vi "Handle Error.vi"(8 "error in (no error)":errorcluster, 11 "UI Actor in":refnum<class "UI Actor.lvclass">) -> (0 "error out":errorcluster, 2 "stop actor?":bool=TRUE, 3 "UI Actor out":refnum<class "UI Actor.lvclass">)   [LabVIEW 2024, in "UI Actor.lvlib" / "UI Actor.lvclass"]
doc: "<p>(<strong>Filename</strong>: <span class=\"dnl\">Actor Framework.lvlib:Actor.lvclass:Handle Error.vi</span>)</p>\n<p>Defines how the actor handles an error that occurred while processing a message. By default, this method does nothing except stop the actor.</p>"
uses:
  UI Actor.lvclass
  UI Actor.lvclass/UI Actor.ctl
  <vilib>/MGI/Panel Manager/Panel Actor/Panel Actor/Panel Actor.lvclass
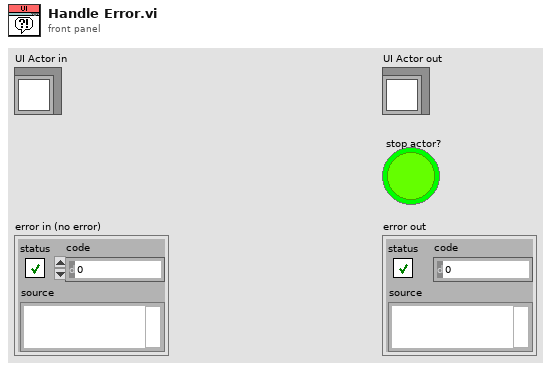
[diagram p1: front panel]
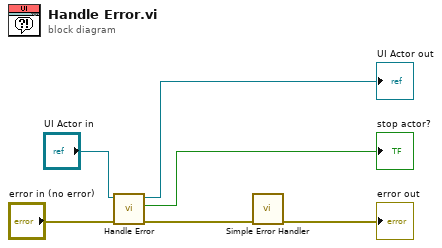
[diagram p0: block diagram]
diagram:
  n1 = call-parent "Handle Error.vi"("error in (no error)"="error in (no error)", "Actor in"="UI Actor in") -> ("error out"=w2:errorcluster, "stop actor?"=→"stop actor?":bool, "Actor out"=→"UI Actor out":refnum<class "UI Actor.lvclass">)  [unwired: 7 in]
  n2 = call <vilib>:"Simple Error Handler.vi"("error in (no error)"=w2) -> ("error out"=→"error out":errorcluster)  [unwired: 4 in, 4 out]
